vi "decode.vi"() -> (3 "status":bool)   [LabVIEW 2012]
uses:
  G_DATA.vi
  G_SEN.vi
  G_NAV.vi
  G_VEH.vi
  G_LCM.vi
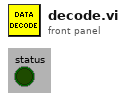
[diagram p1: front panel]
types:
  T1 = cluster{"M6006":string, "M7042":string, "Tcandata":string, "LaserData":string, "SensorData":string, "B_Sencor data 2202":string, "B_object data 2221":string, "Tmobileye":string}
  T2 = cluster{"Header":cluster{"Size of prev messages":u32, "Size of this messages":u32, "Reserved":u8, "DeviceID":u8, "Data type":u16, "NTP time":u64}, "Scan header":cluster{"Scan number":u16, "scanner status":u16, "Sync phase offset":u16, "Scan start time NTP":u64, "Scan end time NTP":u64, "Angle ticks per rotation":u16, "Start angle":dbl, "End angle":dbl, "Scan points":u16, "Mounting position yaw angle ":dbl, "Mounting position pitch angle":dbl, "Mounting position roll angle":dbl, "Mounting position x":dbl, "Mounting position y":dbl, "Mounting position z":dbl, "Reserved":u16}, "Scan points":cluster{"flags":u8, "Echo":u8, "Radial distance":dbl, "Horizontal angle":dbl, "Vertical angle":dbl, "Echo pulse width":u16, "Reserved":u16}[]}
  T3 = enum16{"big-endian, network order", "native, host order", "little-endian"}
  T4 = cluster{"Header":cluster{"Size of prev messages":u32, "Size of this messages":u32, "Reserved":u8, "DeviceID":u8, "Data type":u16, "NTP time":u64}, "Object header":cluster{"NTP time":u64, "Number of objects":u16}, "Objects":cluster{"object":cluster{"Object ID":u16, "Object age ":u16, "Object prediction age":u16, "Relative timestamp":u16, "Reference point X":dbl, "Reference point Y":dbl, "Reference point sigma X":dbl, "Reference point sigma Y":dbl, "Closest point X":dbl, "Closest point Y":dbl, "Bounding box center X":dbl, "Bounding box center Y":dbl, "Bounding box size X":dbl, "Bounding box size Y":dbl, "Object box center X":dbl, "Object box center Y":dbl, "Object box size X":dbl, "Object box size Y":dbl, "Object box orientation":dbl, "Absolute velocity X":dbl, "Absolute velocity Y":dbl, "Absolute velocity sigma X":dbl, "Absolute velocity sigma Y":dbl, "Relative velocity X":dbl, "Relative velocity Y":dbl, "Classification":u16, "Classification age":u16, "Classification certainty":u16, "Number of contour points":u16}, "Contour points":cluster{"Contour points X":dbl, "Contour points Y":dbl}[]}[]}
  T5 = cluster{"global_x":sgl, " global_y":sgl, "yaw":sgl, "objCount":u16, "total":u16}
  T6 = cluster{"GPSTime":dbl, "accel[0]":sgl, "accel[1]":sgl, "accel[2]":sgl, "pqr[0]":sgl, "pqr[1]":sgl, "pqr[2]":sgl, "llh[0]":dbl, "llh[1]":dbl, "llh[2]":dbl, "vel_ned[0]":sgl, "vel_ned[1]":sgl, "vel_ned[2]":sgl, "attitude[0]":sgl, "attitude[1]":sgl, "attitude[2]":sgl, "vel_bxyz[0]":sgl, "vel_bxyz[1]":sgl, "vel_bxyz[2]":sgl, "lcc[0]":sgl, "lcc[1]":sgl, "lcc[2]":sgl, "CovKalman[0]":sgl, "CovKalman[1]":sgl, "CovKalman[2]":sgl, "CovKalman[3]":sgl, "CovKalman[4]":sgl, "CovKalman[5]":sgl, "llh_GPS[0]":sgl, "llh_GPS[1]":sgl, "llh_GPS[2]":sgl, "vel_GPS[0]":sgl, "vel_GPS[1]":sgl, "vel_GPS[2]":sgl, "heading_Magnetic":sgl, "heading_GPS":sgl, "GPSStatus":u16, "FailureCode":u16, "DataChecksum":u16}
  T7 = cluster{"sop1":u8, "sop2":u8, "sop3":u8, "header_length":u8, "number":u16, "type":u8, "port_address":u8, "length":u16, "sequence":u16, "idle":u8, "gps_stat":u8, "gps_week":u16, "millisecs":u32, "status":u32, "crc":u16, "version":u16}
  T8 = cluster{"sol_stat":u32, "pos_type":u32, "lat":dbl, "lon":dbl, "hgt":dbl, "und":sgl, "datum_id":i32, "latdev":sgl, "londev":sgl, "hgtdev":sgl, "ref_station_id 0":i8, "ref_station_id 1":i8, "ref_station_id 2":i8, "ref_station_id 3":i8, "lag":sgl, "age":sgl, "sats":u8, "gps_l1_ranges":u8, "gps_l1_mask_ranges":u8, "gps_l2_mask_ranges":u8, "reserved":i8, "ext_sol_stat":u8, "reserved2":u8, "sig_mask":u8}
  T9 = cluster{"Steer_input":dbl, "Steer_output":dbl, "VS_des":dbl, "VS_can":dbl, "heading":dbl, "auto":bool, "run":bool, "x":dbl, "y":dbl}
  T10 = cluster{"Steer_input":dbl, "Steer_output":dbl, "VS_can":dbl, "auto":bool, "run":bool}
  T11 = cluster{"hash":i64, "utime":i64, "x":dbl, "y":dbl, "h":dbl}
  T12 = cluster{"hash":i64, "utime":i64, "lat":dbl, "long":dbl}
  T13 = cluster{"connection ID":refnum<k16>, "net address":u32, "port":u16}
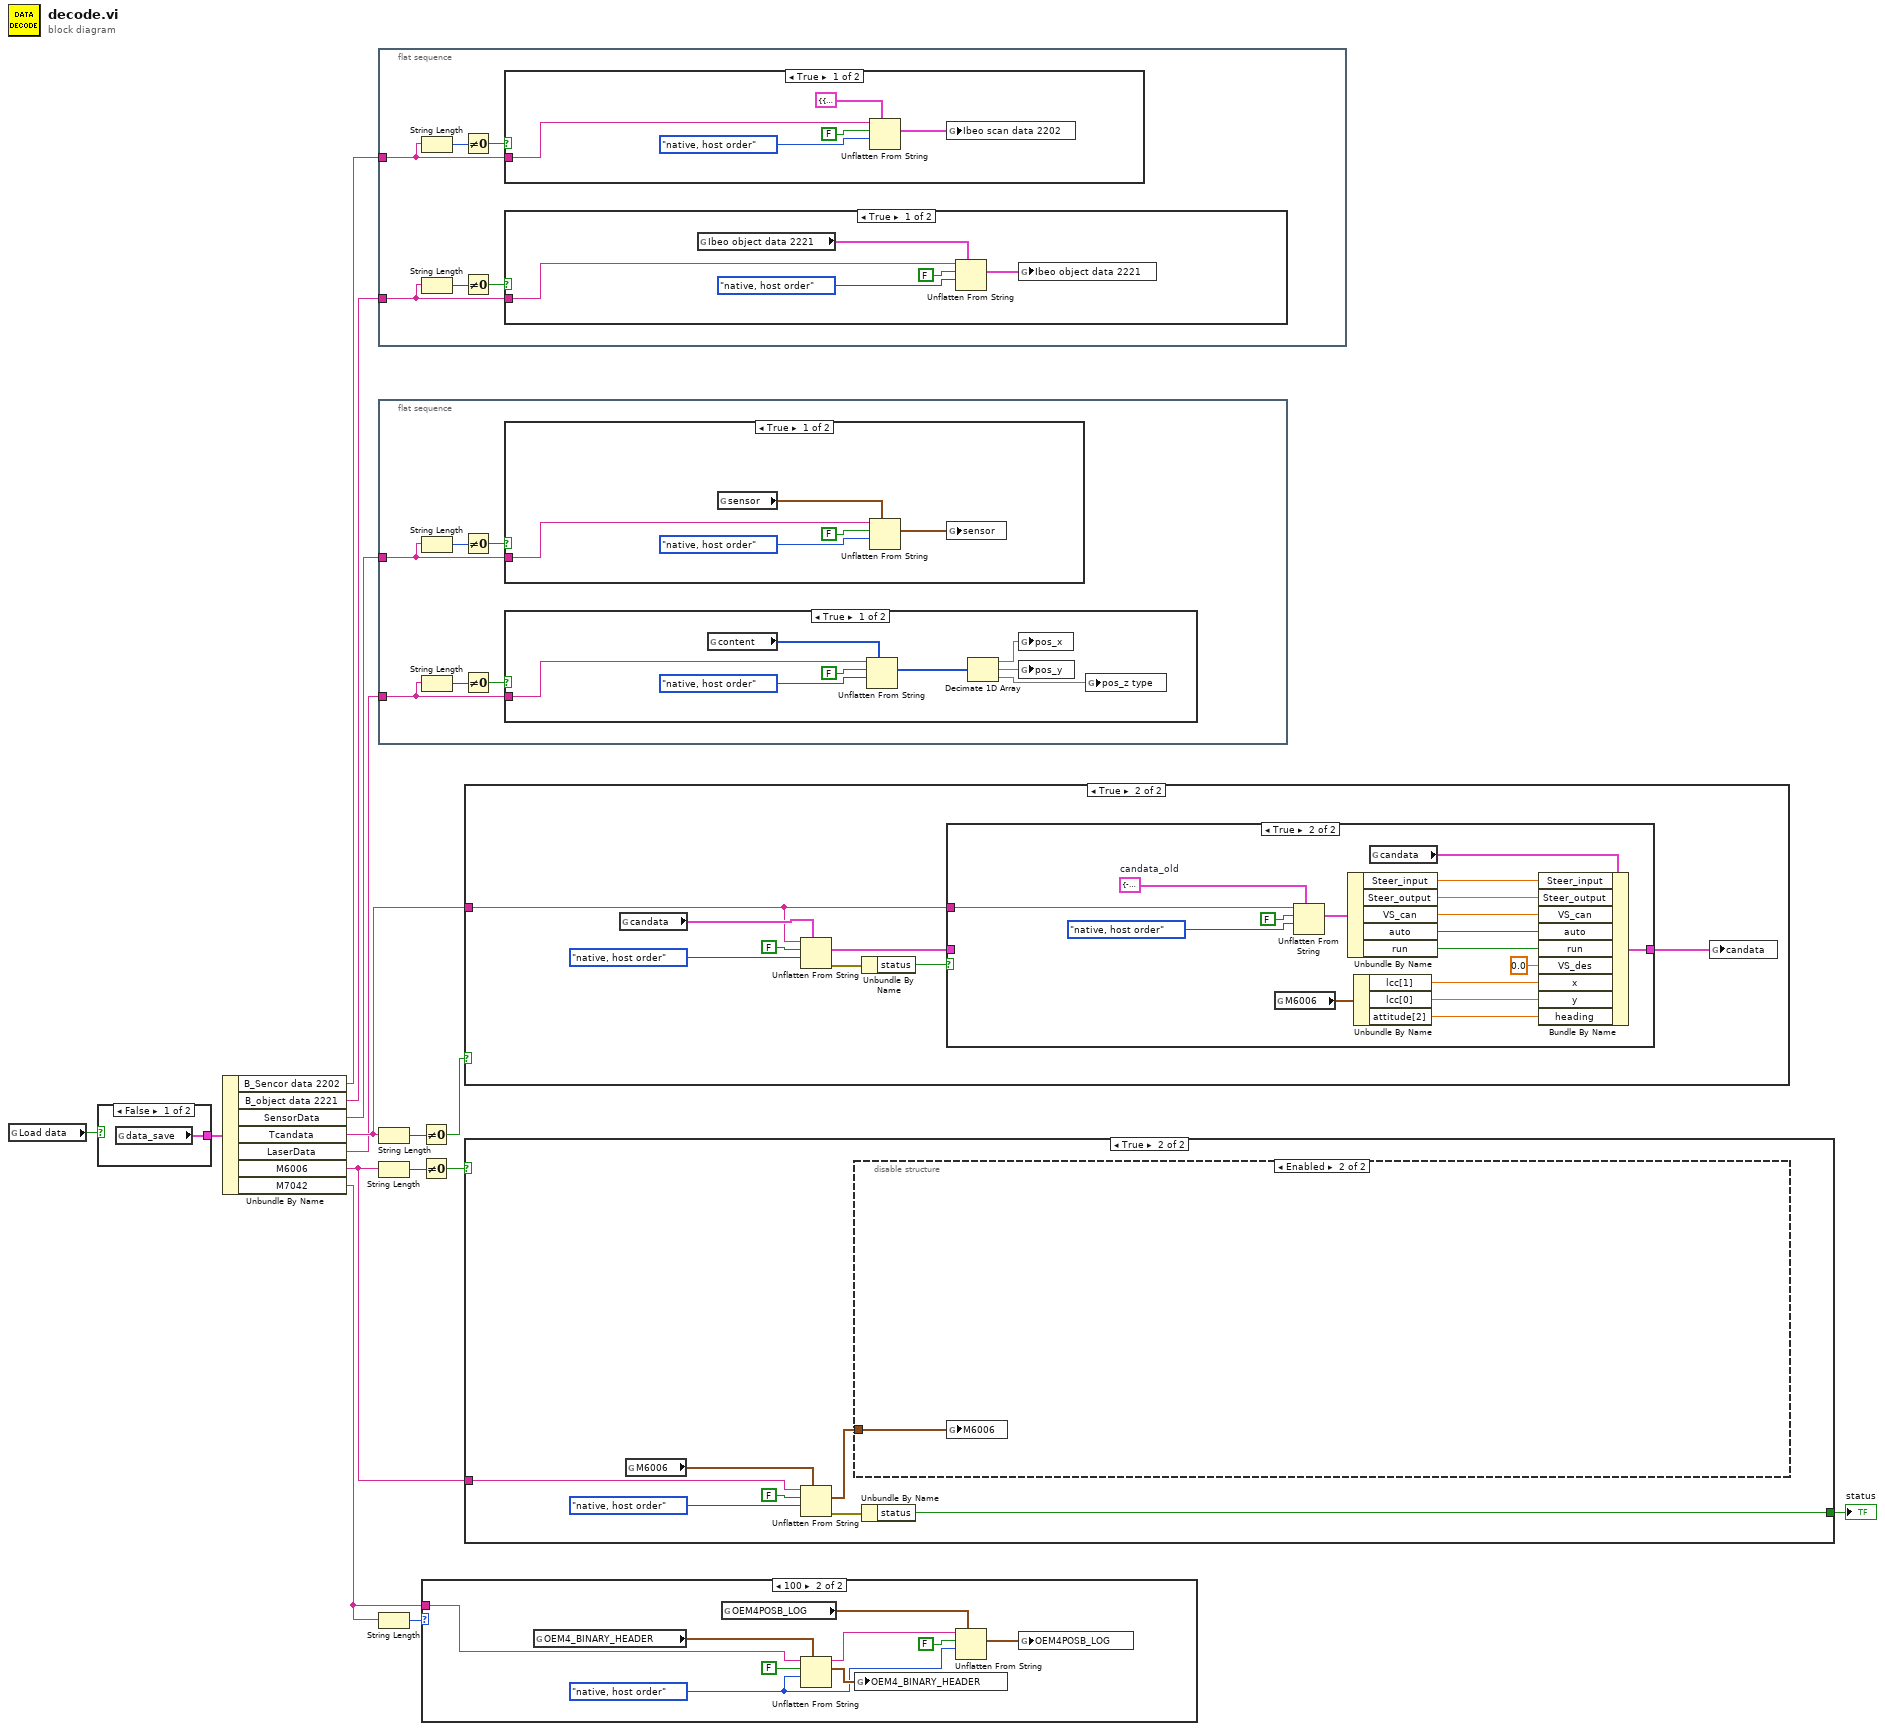
[diagram p0: block diagram]
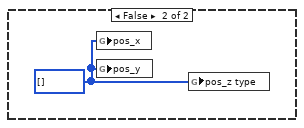
[diagram p2: hidden frame]
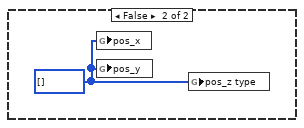
[diagram p3: hidden frame]
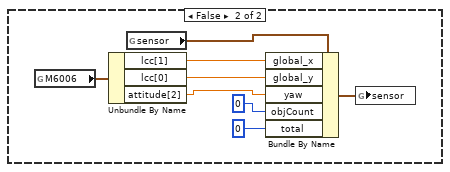
[diagram p4: hidden frame]
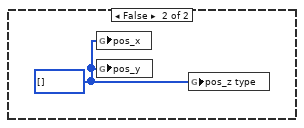
[diagram p5: hidden frame]
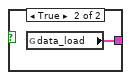
[diagram p6: hidden frame]
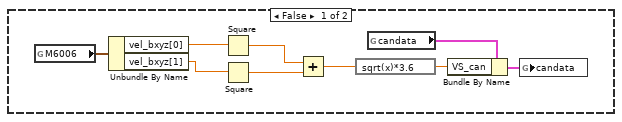
[diagram p7: hidden frame]
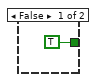
[diagram p10: hidden frame]
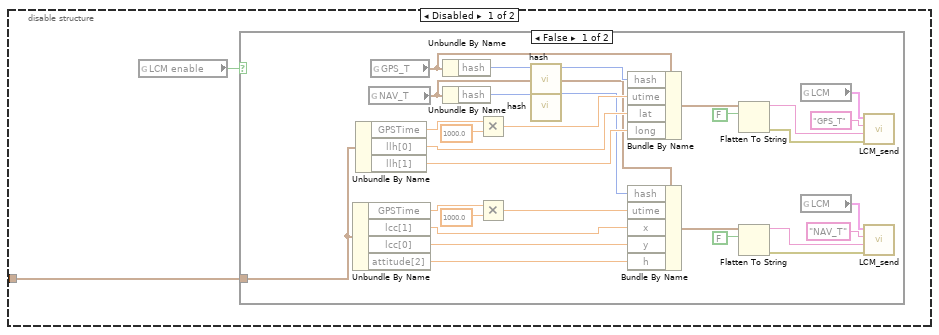
[diagram p11: hidden frame]
diagram:
  n1 = global read "G_DATA.vi" "Load data"() -> (w4:bool)
  n2 = case shown="False" w4 {
    tunnel: [w16 w17] -> w10
    frame False {
      n3 = global read "G_DATA.vi" "data_save"() -> (w16:T1)
    }
    frame True {
      n4 = global read "G_DATA.vi" "data_load"() -> (w17:T1)
    }
  }
  n5 = Unbundle By Name(w10) -> ("B_Sencor data 2202"=w1:string, "B_object data 2221"=w2:string, "SensorData"=w9:string, "Tcandata"=w8:string, "LaserData"=w7:string, "M6006"=w6:string, "M7042"=w5:string)
  n6 = flat-sequence {
    tunnel: w2 -> [w19]
    tunnel: w1 -> [w18]
    frame #0 {
      n7 = String Length(string=w18) -> (length=w21:i32)
      n8 = String Length(string=w19) -> (length=w22:i32)
      n9 = Not Equal To 0?(x=w21) -> (x != 0?=w20:bool)
      n10 = Not Equal To 0?(x=w22) -> (x != 0?=w23:bool)
      n11 = case shown="True" w20 {
        tunnel: w18 -> [w28 _]
        frame True {
          n12 = Unflatten From String(type=T2 {"Header"={"Size of prev messages"=0, "Size of this messages"=0, "Reserved"=0, "DeviceID"=0, "Data type"=0, "NTP time"=0}, "Scan header"={"Scan number"=0, "scanner status"=0, "Sync phase offset"=0, "Scan start time NTP"=0, "Scan end time NTP"=0, "Angle ticks per rotation"=0, "Start angle"=0.0, "End angle"=0.0, "Scan points"=0, "Mounting position yaw angle "=0.0, "Mounting position pitch angle"=0.0, "Mounting position roll angle"=0.0, "Mounting position x"=0.0, "Mounting position y"=0.0, "Mounting position z"=0.0, "Reserved"=0}, "Scan points"=[]} ("output cluster"), binary string=w28, data includes array or string size? (T)=FALSE, byte order (0:big-endian, network order)=T3."native, host order") -> (value=w25:T2)  [unwired: 1 in, 2 out]
          n13 = global write "G_SEN.vi" "Ibeo scan data 2202"(w25) -> ()
        }
        frame False {
          w29 = u16[] [] ("position")
          n14 = global write "G_SEN.vi" "pos_x"(w29) -> ()
          n15 = global write "G_SEN.vi" "pos_y"(w29) -> ()
          n16 = global write "G_SEN.vi" "pos_z type"(w29) -> ()
        }
      }
      n17 = case shown="True" w23 {
        tunnel: w19 -> [w34 _]
        frame True {
          n18 = global read "G_SEN.vi" "Ibeo object data 2221"() -> (w31:T4)
          n19 = Unflatten From String(type=w31, binary string=w34, data includes array or string size? (T)=FALSE, byte order (0:big-endian, network order)=T3."native, host order") -> (value=w30:T4)  [unwired: 1 in, 2 out]
          n20 = global write "G_SEN.vi" "Ibeo object data 2221"(w30) -> ()
        }
        frame False {
          w35 = u16[] [] ("position")
          n21 = global write "G_SEN.vi" "pos_x"(w35) -> ()
          n22 = global write "G_SEN.vi" "pos_y"(w35) -> ()
          n23 = global write "G_SEN.vi" "pos_z type"(w35) -> ()
        }
      }
    }
  }
  n24 = flat-sequence {
    tunnel: w9 -> [w37]
    tunnel: w7 -> [w36]
    frame #0 {
      n25 = String Length(string=w37) -> (length=w39:i32)
      n26 = String Length(string=w36) -> (length=w41:i32)
      n27 = Not Equal To 0?(x=w39) -> (x != 0?=w38:bool)
      n28 = Not Equal To 0?(x=w41) -> (x != 0?=w40:bool)
      n29 = case shown="True" w38 {
        tunnel: w37 -> [w45 _]
        frame True {
          n30 = global read "G_SEN.vi" "sensor"() -> (w46:T5)
          n31 = Unflatten From String(type=w46, binary string=w45, data includes array or string size? (T)=FALSE, byte order (0:big-endian, network order)=T3."native, host order") -> (value=w42:T5)  [unwired: 1 in, 2 out]
          n32 = global write "G_SEN.vi" "sensor"(w42) -> ()
        }
        frame False {
          n33 = global read "G_NAV.vi" "M6006"() -> (w54:T6)
          n34 = Unbundle By Name(w54) -> ("lcc[1]"=w52:sgl, "lcc[0]"=w51:sgl, "attitude[2]"=w50:sgl)
          n35 = global read "G_SEN.vi" "sensor"() -> (w53:T5)
          n36 = Bundle By Name(cluster=w53, "global_x"=w52, "global_y"=w51, "yaw"=w50, "objCount"=u16 0, "total"=u16 0) -> (w47:T5)
          n37 = global write "G_SEN.vi" "sensor"(w47) -> ()
        }
      }
      n38 = case shown="True" w40 {
        tunnel: w36 -> [w61 _]
        frame True {
          n39 = global read "G_SEN.vi" "content"() -> (w62:u16[])
          n40 = Unflatten From String(type=w62, binary string=w61, data includes array or string size? (T)=FALSE, byte order (0:big-endian, network order)=T3."native, host order") -> (value=w55:u16[])  [unwired: 1 in, 2 out]
          n41 = Decimate 1D Array(w55) -> (w56:u16[], w58:u16[], w57:u16[])
          n42 = global write "G_SEN.vi" "pos_x"(w56) -> ()
          n43 = global write "G_SEN.vi" "pos_y"(w58) -> ()
          n44 = global write "G_SEN.vi" "pos_z type"(w57) -> ()
        }
        frame False {
          w63 = u16[] [] ("position")
          n45 = global write "G_SEN.vi" "pos_x"(w63) -> ()
          n46 = global write "G_SEN.vi" "pos_y"(w63) -> ()
          n47 = global write "G_SEN.vi" "pos_z type"(w63) -> ()
        }
      }
    }
  }
  n48 = String Length(string=w8) -> (length=w11:i32)
  n49 = String Length(string=w6) -> (length=w15:i32)
  n50 = String Length(string=w5) -> (length=w13:i32)
  n51 = Not Equal To 0?(x=w11) -> (x != 0?=w12:bool)
  n52 = Not Equal To 0?(x=w15) -> (x != 0?=w14:bool)
  n53 = case shown="100" w13 {
    tunnel: w5 -> [_ w69]
    frame 0, Default {
    }
    frame 100 {
      w66 = T3."native, host order" ("byte order (0:big-endian, network order)")
      n54 = global read "G_NAV.vi" "OEM4_BINARY_HEADER"() -> (w70:T7)
      n55 = global read "G_NAV.vi" "OEM4POSB_LOG"() -> (w64:T8)
      n56 = Unflatten From String(type=w70, binary string=w69, data includes array or string size? (T)=FALSE, byte order (0:big-endian, network order)=w66) -> (rest of the binary string=w68:string, value=w71:T7)  [unwired: 1 in, 1 out]
      n57 = global write "G_NAV.vi" "OEM4_BINARY_HEADER"(w71) -> ()
      n58 = Unflatten From String(type=w64, binary string=w68, data includes array or string size? (T)=FALSE, byte order (0:big-endian, network order)=w66) -> (value=w65:T8)  [unwired: 1 in, 2 out]
      n59 = global write "G_NAV.vi" "OEM4POSB_LOG"(w65) -> ()
    }
  }
  n60 = case shown="True" w12 {
    tunnel: w8 -> [_ w84]
    frame False {
      n61 = global read "G_NAV.vi" "M6006"() -> (w81:T6)
      n62 = Unbundle By Name(w81) -> ("vel_bxyz[0]"=w80:sgl, "vel_bxyz[1]"=w79:sgl)
      n63 = Square(x=w80) -> (x^2=w78:sgl)
      n64 = Square(x=w79) -> (x^2=w77:sgl)
      n65 = Add(x=w78, y=w77) -> (x+y=w76:sgl)
      n66 = expression code="sqrt(x)*3.6"(w76) -> (w74:sgl)
      n67 = global read "G_VEH.vi" "candata"() -> (w73:T9)
      n68 = Bundle By Name(cluster=w73, "VS_can"=w74) -> (w75:T9)
      n69 = global write "G_VEH.vi" "candata"(w75) -> ()
    }
    frame True {
      n70 = global read "G_VEH.vi" "candata"() -> (w87:T9)
      n71 = Unflatten From String(type=w87, binary string=w84, data includes array or string size? (T)=FALSE, byte order (0:big-endian, network order)=T3."native, host order") -> (value=w83:T9, error out=w86:errorcluster)  [unwired: 1 in, 1 out]
      n72 = Unbundle By Name(w86) -> ("status"=w85:bool)
      n73 = case shown="True" w85 {
        tunnel: w84 -> [_ w104]
        tunnel: w83 -> [w90 _]
        tunnel: [w90 w100] -> w82
        frame False {
        }
        frame True {
          w107 = T10 {"Steer_input"=-119.00362066056654, "Steer_output"=-0.0, "VS_can"=0.0, "auto"=FALSE, "run"=FALSE}  # candata_old
          n74 = global read "G_NAV.vi" "M6006"() -> (w99:T6)
          n75 = Unflatten From String(type=w107, binary string=w104, data includes array or string size? (T)=FALSE, byte order (0:big-endian, network order)=T3."native, host order") -> (value=w103:T10)  [unwired: 1 in, 2 out]
          n76 = Unbundle By Name(w103) -> ("Steer_input"=w96:dbl, "Steer_output"=w95:dbl, "VS_can"=w101:dbl, "auto"=w98:bool, "run"=w97:bool)
          n77 = Unbundle By Name(w99) -> ("lcc[1]"=w93:sgl, "lcc[0]"=w92:sgl, "attitude[2]"=w91:sgl)
          n78 = global read "G_VEH.vi" "candata"() -> (w102:T9)
          n79 = Bundle By Name(cluster=w102, "Steer_input"=w96, "Steer_output"=w95, "VS_can"=w101, "auto"=w98, "run"=w97, "VS_des"=0.0, "x"=w93, "y"=w92, "heading"=w91) -> (w100:T9)
        }
      }
      n80 = global write "G_VEH.vi" "candata"(w82) -> ()
    }
  }
  n81 = case shown="True" w14 {
    tunnel: w6 -> [_ w112]
    tunnel: [TRUE ("status") w110] -> w3
    frame False {
    }
    frame True {
      n82 = global read "G_NAV.vi" "M6006"() -> (w113:T6)
      n83 = Unflatten From String(type=w113, binary string=w112, data includes array or string size? (T)=FALSE, byte order (0:big-endian, network order)=T3."native, host order") -> (value=w109:T6, error out=w111:errorcluster)  [unwired: 1 in, 1 out]
      n84 = disable-structure shown="Enabled" {
        disable-tunnel: w109 -> [w117 w148]
        frame Disabled {
          n85 = global read "G_LCM.vi" "LCM enable"() -> (w116:bool)
          n86 = case shown="False" w116 {
            tunnel: w117 -> [w119 _]
            frame False {
              n87 = Unbundle By Name(w119) -> ("GPSTime"=w123:dbl, "lcc[1]"=w126:sgl, "lcc[0]"=w127:sgl, "attitude[2]"=w118:sgl)
              n88 = Unbundle By Name(w119) -> ("GPSTime"=w144:dbl, "llh[0]"=w141:dbl, "llh[1]"=w140:dbl)
              n89 = global read "G_LCM.vi" "NAV_T"() -> (w120:T11)
              n90 = global read "G_LCM.vi" "GPS_T"() -> (w147:T12)
              n91 = Unbundle By Name(w147) -> ("hash"=w146:i64)
              n92 = Unbundle By Name(w120) -> ("hash"=w121:i64)
              n93 = Multiply(x=w144, y=1000.0) -> (x*y=w142:dbl)
              n94 = Multiply(x=w123, y=1000.0) -> (x*y=w125:dbl)
              n95 = call "hash.vi"("input"=w146) -> ("output"=w145:i64)  [unwired: 10 in]
              n96 = call "hash.vi"("input"=w121) -> ("output"=w122:i64)  [unwired: 10 in]
              n97 = Bundle By Name(cluster=w147, "hash"=w145, "utime"=w142, "lat"=w141, "long"=w140) -> (w134:T12)
              n98 = Bundle By Name(cluster=w120, "hash"=w122, "utime"=w125, "x"=w126, "y"=w127, "h"=w118) -> (w133:T11)
              n99 = Flatten To String(anything=w134, prepend array or string size? (T)=FALSE) -> (data string=w135:string, error out=w139:errorcluster)  [unwired: 2 in, 1 out]
              n100 = Flatten To String(anything=w133, prepend array or string size? (T)=FALSE) -> (data string=w132:string, error out=w128:errorcluster)  [unwired: 2 in, 1 out]
              n101 = global read "G_LCM.vi" "LCM"() -> (w138:T13)
              n102 = global read "G_LCM.vi" "LCM"() -> (w129:T13)
              n103 = call "LCM_send.vi"("error in (no error)"=w139, "DATA"=w135, "ID"="GPS_T", "LCM"=w138) -> ()  [unwired: 5 in, 3 out]
              n104 = call "LCM_send.vi"("error in (no error)"=w128, "DATA"=w132, "ID"="NAV_T", "LCM"=w129) -> ()  [unwired: 5 in, 3 out]
            }
            frame True {
            }
          }
        }
        frame Enabled {
          n105 = global write "G_NAV.vi" "M6006"(w148) -> ()
        }
      }
      n106 = Unbundle By Name(w111) -> ("status"=w110:bool)
    }
  }
  "status" <- w3
